vi "Read_Camram_Example_IMAQ.vi"() -> ()   [LabVIEW 2019]
uses:
  camera/Camera.lvclass
panel:
  out "rawImage":u16[][](array[numeric])
  out "Image":T1(plugin-control)
  in  "data_format":T2(ring)=enum."Mono16"
  in  "Image Index":u32 max=2
  out "Recorded Images":u32
  in  "Quit":bool
  in  "roiY1":u64=2 min=2 max=2016 step=1
  in  "roiX1":u64=2 min=2 max=2016 step=1
  in  "roiY0":u64=1 min=1 max=2015 step=1
  in  "roiX0":u64=1 min=1 max=2015 step=1
  out "Image Height":u16
  out "Image Width":u16
  in  "segment":u16=3 caption="Segment" min=1 max=4
  out "Error":errorcluster {"code" format="%x"}
  # "This example shows for cameras with internal memory how to read images from ram, already available from a previous record\nIt is a good starting point for writing own applications.\nBut it will not be fail save, i.e. doesnt react on errors, just handles them forward to the end\n\nUsage:\nSelect the segment you want to read from before you start the program. \nThis segment must already contain images, otherwise the read will fail\nOnce started, the camera class will be initialized and images will be recorded automatically.\nWhen acquisition has finished you can address the images and set a certain roi \nTo finish the program click on quit application, this will force fan exit of the camera class"
  # "pco.labview"
  # "Camera Setup"
  # "Recording Control"
  # "Parameters for image readout"
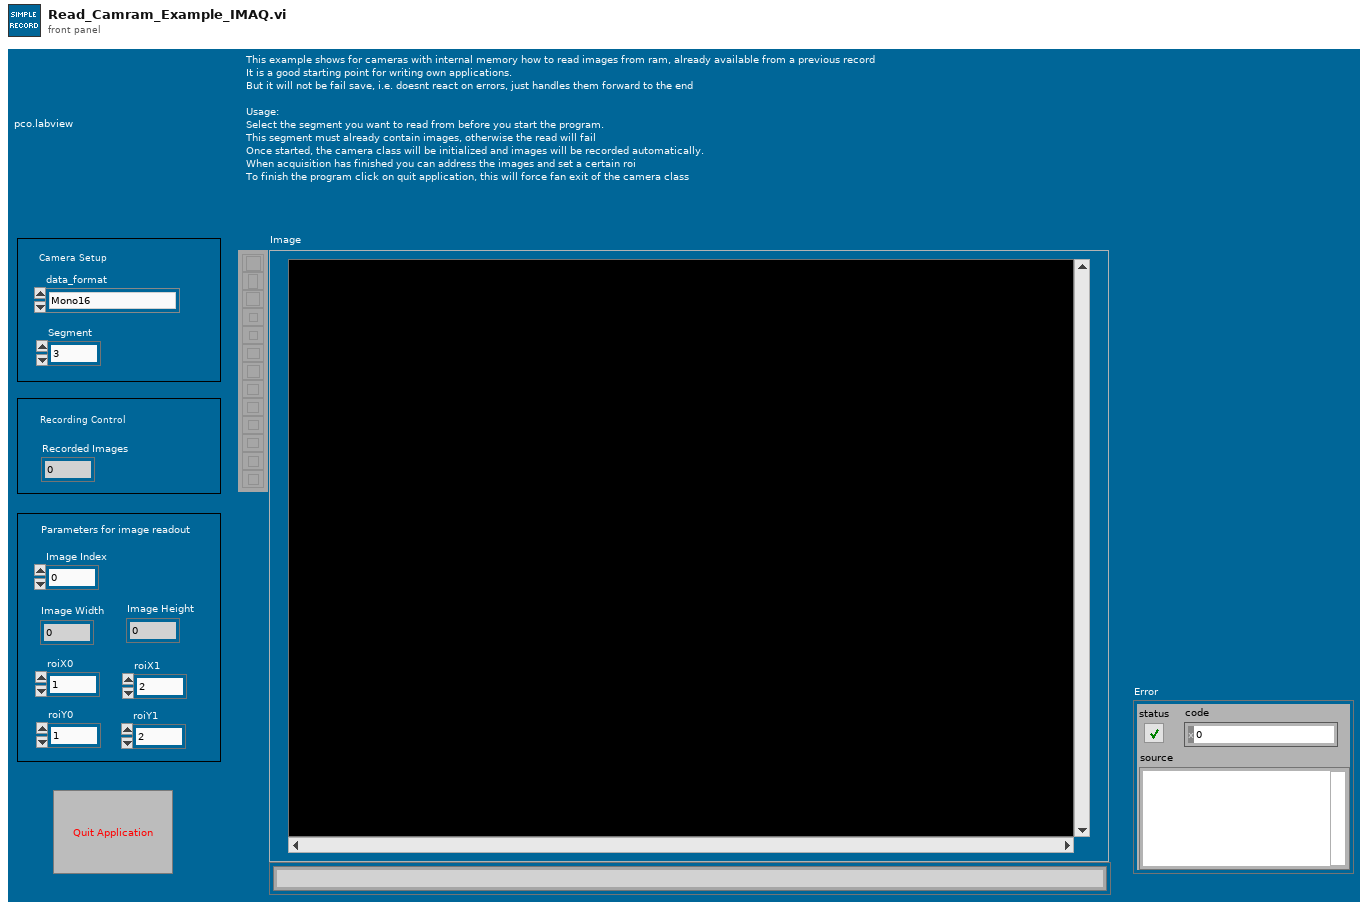
[diagram p1: front panel]
types:
  T1 = typedef "IMAQ Image.ctl" = refnum<image>
  T2 = enum16{"Undefined", "Mono8", "Mono16", "BGRA8", "RGBA8", "BGRA16", "RGBA16", "CompressedMono8"}
  T3 = enum8{"Enabled", "Disabled", "Disabled and Grayed Out"}
  T4 = cluster{"serial":u32, "type":u16, "sub_type":u16, "interface_type":u16, "bit_resolution":u16, "min_exposure_time_s":dbl, "max_exposure_time_s":dbl, "min_exposure_step_s":dbl, "min_delay_time_s":dbl, "max_delay_time_s":dbl, "min_delay_step_s":dbl, "min_width":u64, "min_height":u64, "max_width":u64, "max_height":u64, "roi_step_horz":u64, "roi_step_vert":u64, "roi_symmetric_horz":bool, "roi_symmetric_vert":bool, "has_timestamp_mode":bool, "has_timestamp_mode_ascii_only":bool, "pixelrate_vec":u32[], "conversion_factor_vec":sgl[], "has_trigger_mode_extexpctrl":bool, "has_acquire_mode":bool, "has_ext_acquire_mode":bool, "has_metadata_mode":bool, "has_ram":bool, "binning_horz_vec":u16[], "binning_vert_vec":u16[], "has_average_binning":bool, "pixel_format_vec":u32[]}
  T5 = typedef "Image Type" = u32
  T6 = typedef "Camera.lvclass/binning.ctl" = cluster{"vert":u16, "horz":u16, "mode":u16}
  T7 = cluster{"exposure_time_s":dbl, "delay_time_s":dbl, "roi":cluster{"x0":u64, "y0":u64, "x1":u64, "y1":u64}, "timestamp_mode":u16, "pixelrate":u32, "conversion_factor":sgl, "trigger_mode":u16, "acquire_mode":u16, "acquire_sequence_number":u32, "metadata_mode":u16, "noisefilter_mode":u16, "pixel_format":u32, "binning":T6, "auto_exposure":cluster{"region":u16, "min_exposure_s":dbl, "max_exposure_s":dbl}}
  T8 = cluster{"Plane 4 (alpha)":u16, "Plane 1 (Red)":u16, "Plane 2 (Green)":u16, "Plane 3 (Blue)":u16}[][]
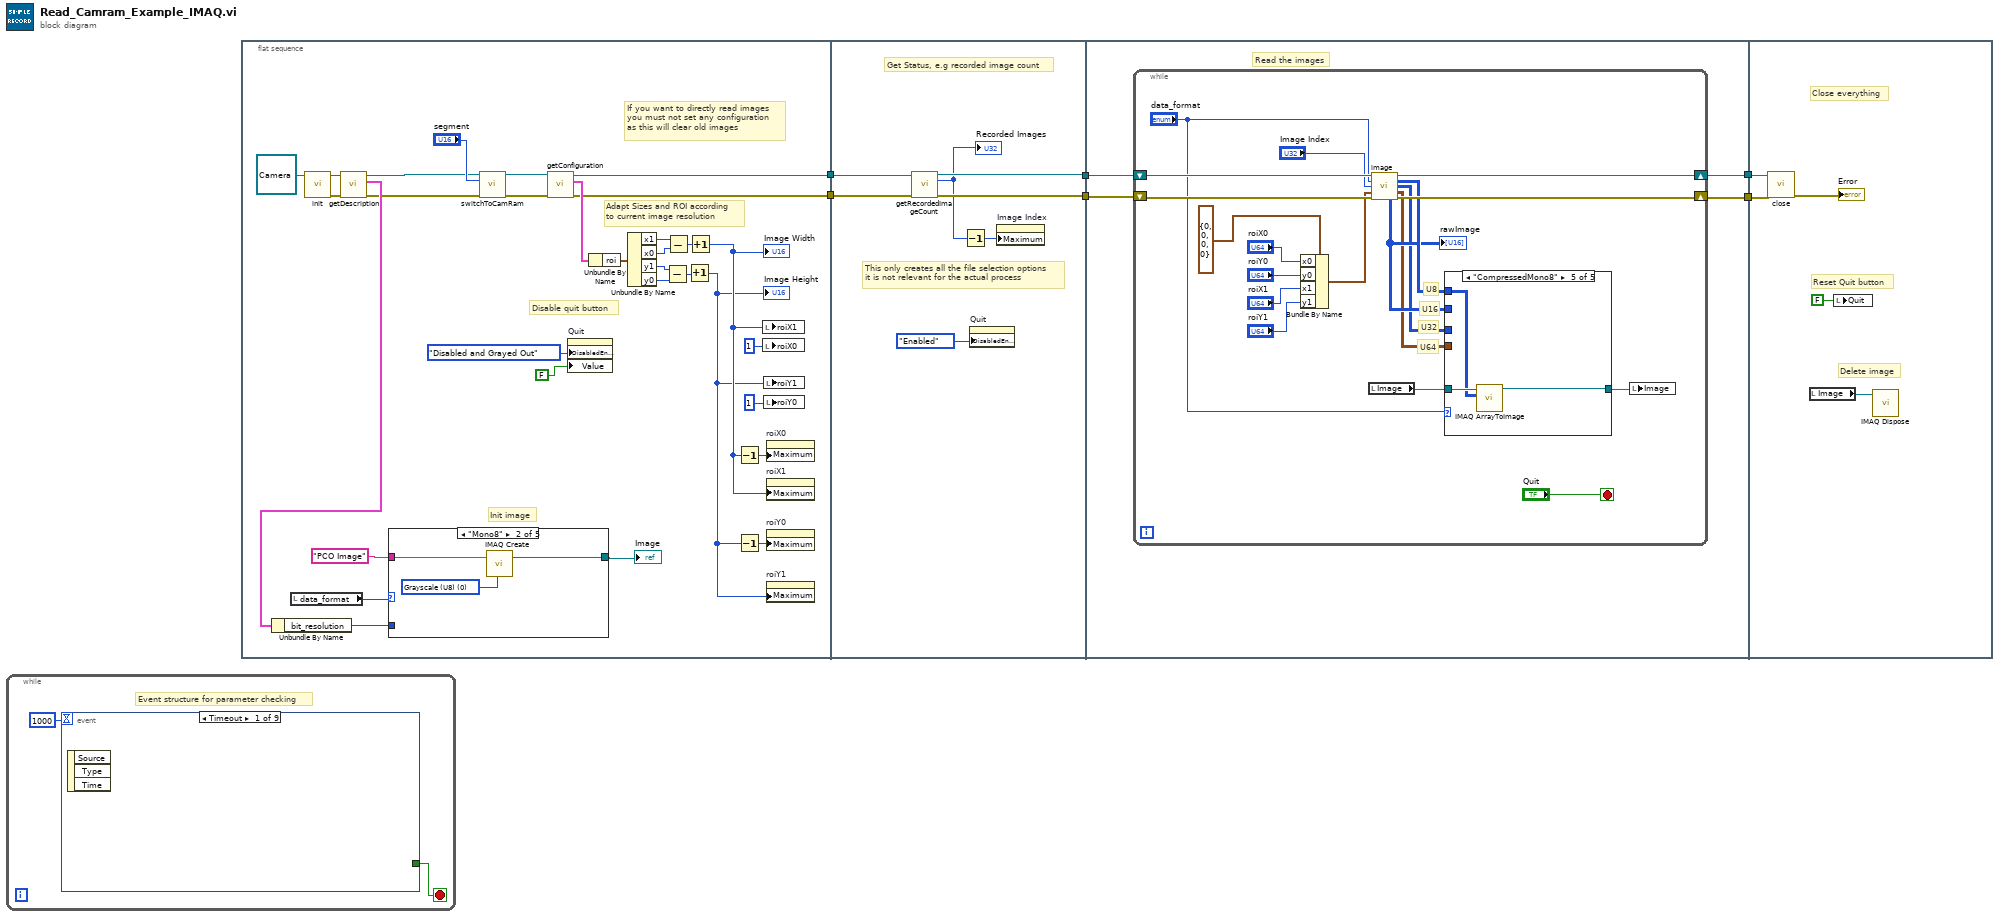
[diagram p0: block diagram]
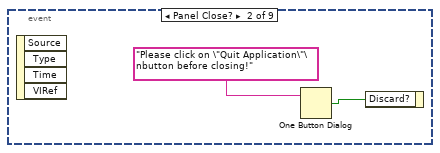
[diagram p2: hidden frame]
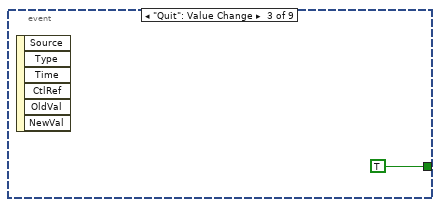
[diagram p3: hidden frame]
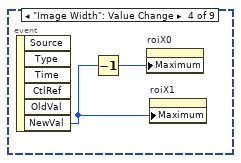
[diagram p4: hidden frame]
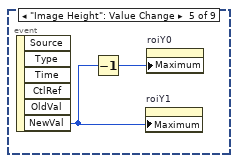
[diagram p5: hidden frame]
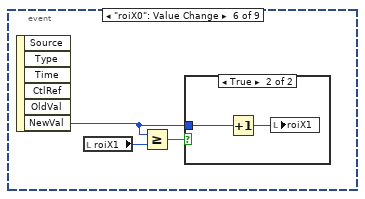
[diagram p6: hidden frame]
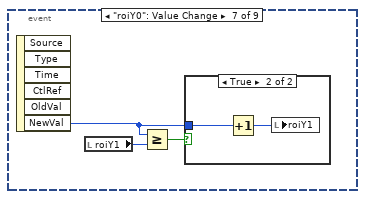
[diagram p8: hidden frame]
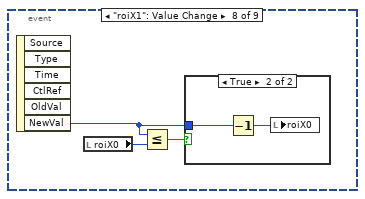
[diagram p10: hidden frame]
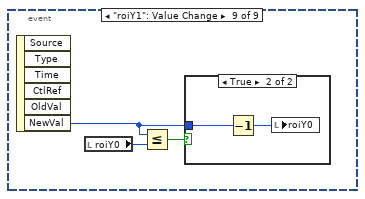
[diagram p12: hidden frame]
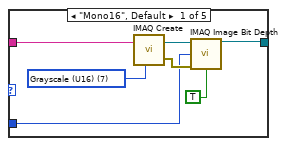
[diagram p14: hidden frame]
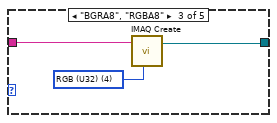
[diagram p15: hidden frame]
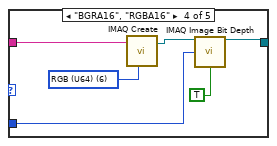
[diagram p16: hidden frame]
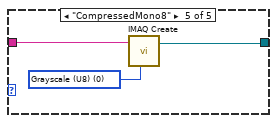
[diagram p17: hidden frame]
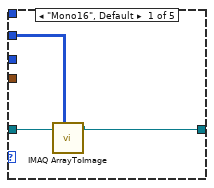
[diagram p18: hidden frame]
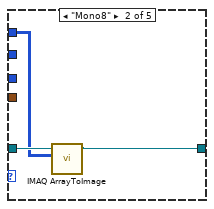
[diagram p19: hidden frame]
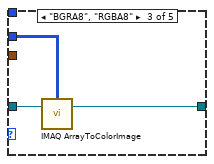
[diagram p20: hidden frame]
diagram:
  n1 = while {
    stop <- w7 stop-if-true
    # "Event structure for parameter checking"
    n2 = event shown="[0] Timeout" {
      selector: _ -> [_ _ _ _ _ _ _ _ _]
      dyn-events: _ -> [_ _ _ _ _ _ _ _ _]
      timeout: 1000 -> [_ _ _ _ _ _ _ _ _]
      tunnel: [_ _ TRUE _ _ _ _ _ _] -> w7
      event Timeout {
        n3 = event-data() -> ()  [unwired: 1 in, 3 out]
      }
      event Panel Close? {
        n4 = event-data() -> ()  [unwired: 1 in, 4 out]
        n5 = One Button Dialog(message="Please click on \"Quit Application\"\nbutton before closing!") -> (true=w9:bool)  [unwired: 1 in]
        n6 = event-data("Discard?"=w9) -> ()  [unwired: 1 in, 1 out]
      }
      event "Quit": Value Change {
        n7 = event-data() -> ()  [unwired: 1 in, 6 out]
      }
      event "Image Width": Value Change {
        n8 = event-data() -> ("NewVal"=w12:u16)  [unwired: 1 in, 5 out]
        n9 = Decrement(x=w12) -> (x-1=w13:u16)
        n10 = property on="roiX0" class="DigNum (strict)"("Maximum"=w13) -> ()  [unwired: 2 in, 2 out]
        n11 = property on="roiX1" class="DigNum (strict)"("Maximum"=w12) -> ()  [unwired: 2 in, 2 out]
      }
      event "Image Height": Value Change {
        n12 = event-data() -> ("NewVal"=w14:u16)  [unwired: 1 in, 5 out]
        n13 = Decrement(x=w14) -> (x-1=w15:u16)
        n14 = property on="roiY1" class="DigNum (strict)"("Maximum"=w14) -> ()  [unwired: 2 in, 2 out]
        n15 = property on="roiY0" class="DigNum (strict)"("Maximum"=w15) -> ()  [unwired: 2 in, 2 out]
      }
      event "roiX0": Value Change {
        n16 = event-data() -> ("NewVal"=w16:u64)  [unwired: 1 in, 5 out]
        n17 = local read "roiX1"() -> (w18:u64)
        n18 = Greater Or Equal?(x=w16, y=w18) -> (x >= y?=w17:bool)
        n19 = case shown="True" w17 {
          tunnel: w16 -> [_ w20]
          frame False {
          }
          frame True {
            n20 = Increment(x=w20) -> (x+1=w19:u64)
            n21 = local write "roiX1"(w19) -> ()
          }
        }
      }
      event "roiY0": Value Change {
        n22 = event-data() -> ("NewVal"=w21:u64)  [unwired: 1 in, 5 out]
        n23 = local read "roiY1"() -> (w23:u64)
        n24 = Greater Or Equal?(x=w21, y=w23) -> (x >= y?=w22:bool)
        n25 = case shown="True" w22 {
          tunnel: w21 -> [_ w25]
          frame False {
          }
          frame True {
            n26 = Increment(x=w25) -> (x+1=w24:u64)
            n27 = local write "roiY1"(w24) -> ()
          }
        }
      }
      event "roiX1": Value Change {
        n28 = event-data() -> ("NewVal"=w26:u64)  [unwired: 1 in, 5 out]
        n29 = local read "roiX0"() -> (w28:u64)
        n30 = Less Or Equal?(x=w26, y=w28) -> (x <= y?=w27:bool)
        n31 = case shown="True" w27 {
          tunnel: w26 -> [_ w30]
          frame False {
          }
          frame True {
            n32 = Decrement(x=w30) -> (x-1=w29:u64)
            n33 = local write "roiX0"(w29) -> ()
          }
        }
      }
      event "roiY1": Value Change {
        n34 = event-data() -> ("NewVal"=w31:u64)  [unwired: 1 in, 5 out]
        n35 = local read "roiY0"() -> (w33:u64)
        n36 = Less Or Equal?(x=w31, y=w33) -> (x <= y?=w32:bool)
        n37 = case shown="True" w32 {
          tunnel: w31 -> [_ w35]
          frame False {
          }
          frame True {
            n38 = Decrement(x=w35) -> (x-1=w34:u64)
            n39 = local write "roiY0"(w34) -> ()
          }
        }
      }
    }
  }
  n40 = flat-sequence {
    tunnel: [w39] -> w6
    tunnel: [w38] -> w5
    tunnel: [w95] -> w4
    tunnel: [w94] -> w3
    tunnel: w6 -> [w90]
    tunnel: w5 -> [w89]
    tunnel: w4 -> [w98]
    tunnel: w3 -> [w99]
    tunnel: [w97] -> w2
    tunnel: [w96] -> w1
    tunnel: w2 -> [w136]
    tunnel: w1 -> [w135]
    frame #0 {
      # "If you want to directly read images\nyou must not set any configuration\nas this will clear old images"
      # "Init image"
      # "Adapt Sizes and ROI according\nto current image resolution"
      # "Disable quit button"
      n41 = local read "data_format"() -> (w49:T2)
      n42 = call-dynamic "init.vi"("Camera in"=refnum<class "Camera.lvclass"> refnum ("PCOCamera in")) -> ("Camera out"=w45:refnum<class "Camera.lvclass">, "error out"=w46:errorcluster)  [unwired: 8 in]
      n43 = call-dynamic "getDescription.vi"("error in (no error)"=w46, "Camera in"=w45) -> ("error out"=w36:errorcluster, "description"=w44:T4, "Camera out"=w37:refnum<class "Camera.lvclass">)  [unwired: 7 in]
      n44 = Unbundle By Name(w44) -> ("bit_resolution"=w43:u16)
      n45 = case shown="\"Mono8\"" w49 {
        tunnel: "PCO Image" ("Image Name") -> [w72 w76 w78 w84 w87]
        tunnel: [w68 w74 w77 w81 w86] -> w48
        tunnel: w43 -> [w67 _ _ w80 _]
        frame "Mono16", Default {
          w73 = T5 7 items=["Grayscale (U8)", "Grayscale (I16)", "Grayscale (SGL)", "Complex (CSG)", "RGB (U32)", "HSL (U32)", "RGB (U64)", "Grayscale (U16)"] ("Image Type")
          n46 = call "IMAQ Create"("Image Name"=w72, "Image Type"=w73) -> ("New Image"=w70:T1, "error out"=w69:errorcluster)  [unwired: 3 in]
          n47 = call "IMAQ Image Bit Depth"("Image"=w70, "Bit Depth (0)"=w67, "error in (no error)"=w69, "Get/Set Bit Depth? (Set)"=TRUE) -> ("Image Out"=w68:T1)  [unwired: 9 in, 2 out]
        }
        frame "Mono8" {
          w75 = T5 0 items=["Grayscale (U8)", "Grayscale (I16)", "Grayscale (SGL)", "Complex (CSG)", "RGB (U32)", "HSL (U32)", "RGB (U64)", "Grayscale (U16)"] ("Image Type")
          n48 = call "IMAQ Create"("Image Name"=w76, "Image Type"=w75) -> ("New Image"=w74:T1)  [unwired: 3 in, 1 out]
        }
        frame "BGRA8", "RGBA8" {
          w79 = T5 4 items=["Grayscale (U8)", "Grayscale (I16)", "Grayscale (SGL)", "Complex (CSG)", "RGB (U32)", "HSL (U32)", "RGB (U64)", "Grayscale (U16)"] ("Image Type")
          n49 = call "IMAQ Create"("Image Name"=w78, "Image Type"=w79) -> ("New Image"=w77:T1)  [unwired: 3 in, 1 out]
        }
        frame "BGRA16", "RGBA16" {
          w85 = T5 6 items=["Grayscale (U8)", "Grayscale (I16)", "Grayscale (SGL)", "Complex (CSG)", "RGB (U32)", "HSL (U32)", "RGB (U64)", "Grayscale (U16)"] ("Image Type")
          n50 = call "IMAQ Create"("Image Name"=w84, "Image Type"=w85) -> ("New Image"=w82:T1)  [unwired: 3 in, 1 out]
          n51 = call "IMAQ Image Bit Depth"("Image"=w82, "Bit Depth (0)"=w80, "Get/Set Bit Depth? (Set)"=TRUE) -> ("Image Out"=w81:T1)  [unwired: 10 in, 2 out]
        }
        frame "CompressedMono8" {
          w88 = T5 0 items=["Grayscale (U8)", "Grayscale (I16)", "Grayscale (SGL)", "Complex (CSG)", "RGB (U32)", "HSL (U32)", "RGB (U64)", "Grayscale (U16)"] ("Image Type")
          n52 = call "IMAQ Create"("Image Name"=w87, "Image Type"=w88) -> ("New Image"=w86:T1)  [unwired: 3 in, 1 out]
        }
      }
      "Image" <- w48
      n53 = call-dynamic "switchToCamRam.vi"("Camera in"=w37, "segment"="segment", "error in (no error)"=w36) -> ("Camera out"=w42:refnum<class "Camera.lvclass">, "error out"=w41:errorcluster)  [unwired: 11 in]
      n54 = call-dynamic "getConfiguration.vi"("error in (no error)"=w41, "Camera in"=w42) -> ("error out"=w38:errorcluster, "configuration"=w61:T7, "Camera out"=w39:refnum<class "Camera.lvclass">)  [unwired: 7 in]
      n55 = property on="Quit" class="Bool (strict)"("DisabledEnum"=T3."Disabled and Grayed Out" ("Disabled"), "Value"=FALSE ("Stop")) -> ()  [unwired: 2 in, 2 out]
      n56 = Unbundle By Name(w61) -> ("roi"=w60:cluster{"x0":u64, "y0":u64, "x1":u64, "y1":u64})
      n57 = Unbundle By Name(w60) -> ("x1"=w58:u64, "x0"=w59:u64, "y1"=w56:u64, "y0"=w57:u64)
      n58 = Subtract(x=w56, y=w57) -> (x-y=w54:u64)
      n59 = Subtract(x=w58, y=w59) -> (x-y=w55:u64)
      n60 = Increment(x=w54) -> (x+1=w52:u64)
      "Image Height" <- w52
      n61 = Increment(x=w55) -> (x+1=w53:u64)
      "Image Width" <- w53
      n62 = Decrement(x=w53) -> (x-1=w63:u64)
      n63 = Decrement(x=w52) -> (x-1=w62:u64)
      n64 = local write "roiX1"(w53) -> ()
      n65 = local write "roiX0"(u16 1 ("roiY0")) -> ()
      n66 = local write "roiY1"(w52) -> ()
      n67 = local write "roiY0"(u16 1 ("roiY0")) -> ()
      n68 = property on="roiX0" class="DigNum (strict)"("Maximum"=w63) -> ()  [unwired: 2 in, 2 out]
      n69 = property on="roiX1" class="DigNum (strict)"("Maximum"=w53) -> ()  [unwired: 2 in, 2 out]
      n70 = property on="roiY0" class="DigNum (strict)"("Maximum"=w62) -> ()  [unwired: 2 in, 2 out]
      n71 = property on="roiY1" class="DigNum (strict)"("Maximum"=w52) -> ()  [unwired: 2 in, 2 out]
    }
    frame #1 {
      # "This only creates all the file selection options\nit is not relevant for the actual process"
      # "Get Status, e.g recorded image count"
      n72 = call-dynamic "getRecordedImageCount.vi"("Camera in"=w90, "error in (no error)"=w89) -> ("Camera out"=w95:refnum<class "Camera.lvclass">, "recorded_image_count"=w91:u32, "error out"=w94:errorcluster)  [unwired: 11 in]
      "Recorded Images" <- w91
      n73 = Decrement(x=w91) -> (x-1=w92:u32)
      n74 = property on="Quit" class="Bool (strict)"("DisabledEnum"=T3."Enabled" ("Disabled")) -> ()  [unwired: 2 in, 2 out]
      n75 = property on="Image Index" class="DigNum (strict)"("Maximum"=w92) -> ()  [unwired: 2 in, 2 out]
    }
    frame #2 {
      # "Read the images"
      n76 = while {
        shift-right: [w116] -> w97
        shift-left: w98 -> [w118]
        shift-right: [w111] -> w96
        shift-left: w99 -> [w117]
        stop <- "Quit" stop-if-true
        # "U64"
        # "U32"
        # "U16"
        # "U8"
        n77 = Bundle By Name(cluster=cluster{"x0":u64, "y0":u64, "x1":u64, "y1":u64} {"x0"=0, "y0"=0, "x1"=0, "y1"=0} ("roi"), "x0"="roiX0", "y0"="roiY0", "x1"="roiX1", "y1"="roiY1") -> (w110:cluster{"x0":u64, "y0":u64, "x1":u64, "y1":u64})
        n78 = local read "Image"() -> (w103:T1)
        n79 = call-dynamic "image.vi"("Camera in"=w118, "data_format"="data_format", "image_index"="Image Index", "crop"=w110, "error in (no error)"=w117) -> ("Camera out"=w116:refnum<class "Camera.lvclass">, "image (U8)"=w107:u8[][], "image (U32)"=w105:u32[][], "image (U64)"=w104:T8, "raw_image (U16)"=w106:u16[][], "error out"=w111:errorcluster)  [unwired: 2 in, 3 out]
        "rawImage" <- w106
        n80 = case shown="\"CompressedMono8\"" "data_format" {
          tunnel: w103 -> [w121 w124 w127 w130 w133]
          tunnel: [w119 w122 w126 w128 w132] -> w102
          tunnel: w104 -> [_ _ _ w129 _]
          tunnel: w105 -> [_ _ w125 _ _]
          tunnel: w107 -> [_ w123 _ _ w131]
          tunnel: w106 -> [w120 _ _ _ _]
          frame "Mono16", Default {
            n81 = call "IMAQ ArrayToImage"("Image Pixels (U16)"=w120, "Image"=w121) -> ("Image Out"=w119:T1)  [unwired: 8 in, 1 out]
          }
          frame "Mono8" {
            n82 = call "IMAQ ArrayToImage"("Image Pixels (U8)"=w123, "Image"=w124) -> ("Image Out"=w122:T1)  [unwired: 8 in, 1 out]
          }
          frame "BGRA8", "RGBA8" {
            n83 = call "IMAQ ArrayToColorImage"("Image Pixels (U32)"=w125, "Image"=w127) -> ("Image Out"=w126:T1)  [unwired: 3 in, 1 out]
          }
          frame "BGRA16", "RGBA16" {
            n84 = call "IMAQ ArrayToColorImage"("Image"=w130, "Image Pixels (U64)"=w129) -> ("Image Out"=w128:T1)  [unwired: 3 in, 1 out]
          }
          frame "CompressedMono8" {
            n85 = call "IMAQ ArrayToImage"("Image Pixels (U8)"=w131, "Image"=w133) -> ("Image Out"=w132:T1)  [unwired: 8 in, 1 out]
          }
        }
        n86 = local write "Image"(w102) -> ()
      }
    }
    frame #3 {
      # "Delete image"
      # "Reset Quit button"
      # "Close everything"
      n87 = call-dynamic "close.vi"("error in (no error)"=w135, "Camera in"=w136) -> ("error out"=→"Error":errorcluster)  [unwired: 9 in]
      n88 = local read "Image"() -> (w134:T1)
      n89 = local write "Quit"(FALSE ("Stop")) -> ()
      n90 = call "IMAQ Dispose"("Image"=w134) -> ()  [unwired: 5 in, 1 out]
    }
  }
